vi "Teleop.vi"(0 "Call Context":T2, 1 "Match Info":T1={"Autonomous Elapsed Seconds"=0.0, "TeleOp Elapsed Seconds"=0.0, "Disabled Elapsed Seconds"=0.0, "Visited Autonomous"=FALSE, "Visited TeleOp"=FALSE, "Visited Disabled"=FALSE, "Autonomous Settings"={"Autonomous Style"=enum."Independent", "VI Refnum"=refnum}}) -> ()   [LabVIEW 2017]
doc: "This VI is called for each TeleOp packet received from the DS where the robot is not disabled. It is often used to read from the joysticks and update I/O or to update setpoints for timed control loops. It should complete and return within 20 milliseconds or it may miss DS packets."
uses:
  <vilib>/Rock Robotics/Network Tables/NT Write Numeric Array.vi
  <vilib>/Rock Robotics/Network Tables/NT Write Boolean Array.vi
  <vilib>/Rock Robotics/Network Tables/NT Read Boolean.vi
  <vilib>/Rock Robotics/Network Tables/NT Read Number.vi
  <vilib>/Rock Robotics/WPI/DriverStation/WPI_DriverStationMatch Info.ctl
  <vilib>/Rock Robotics/WPI/DriverStation/WPI_DriverStationDerivedRobotMode.ctl
panel:
  out "Compressor Running":bool
  out "Enabled":bool
  out "Sample Slider 0":dbl(slide) scale=0.0..5.0
  out "Sample Boolean 1":bool
  out "Sample Boolean 0":bool
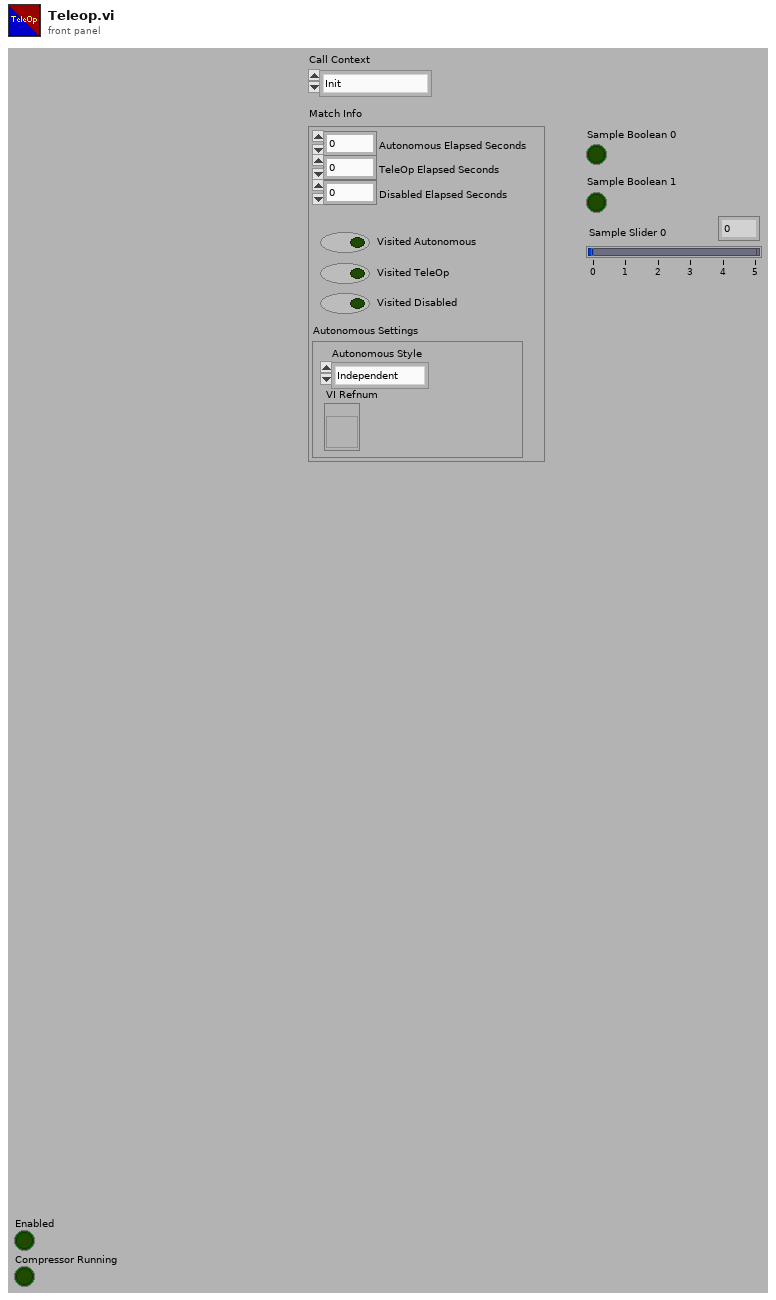
[diagram p1: front panel]
types:
  T1 = typedef "WPI_DriverStationMatch Info.ctl" = cluster{"Autonomous Elapsed Seconds":dbl, "TeleOp Elapsed Seconds":dbl, "Disabled Elapsed Seconds":dbl, "Visited Autonomous":bool, "Visited TeleOp":bool, "Visited Disabled":bool, "Autonomous Settings":cluster{"Autonomous Style":enum16{"Iterative", "Independent"}, "VI Refnum":refnum<vi>}}
  T2 = typedef "WPI_DriverStationDerivedRobotMode.ctl" = enum16{"Init", "Execute", "Stop"}
  T3 = typedef "WPI_CompressorDevRef.ctl" = cluster{"DevStatus":errorcluster, "Pneumatics Control Module":u8}
  T4 = typedef "WPI_JoystickDevRef.ctl" = cluster{"Device":T5}
  T5 = typedef "WPI_JoystickDeviceEnum.ctl" = enum16{"USB 0", "USB 1", "USB 2", "USB 3", "USB 4", "USB 5"}
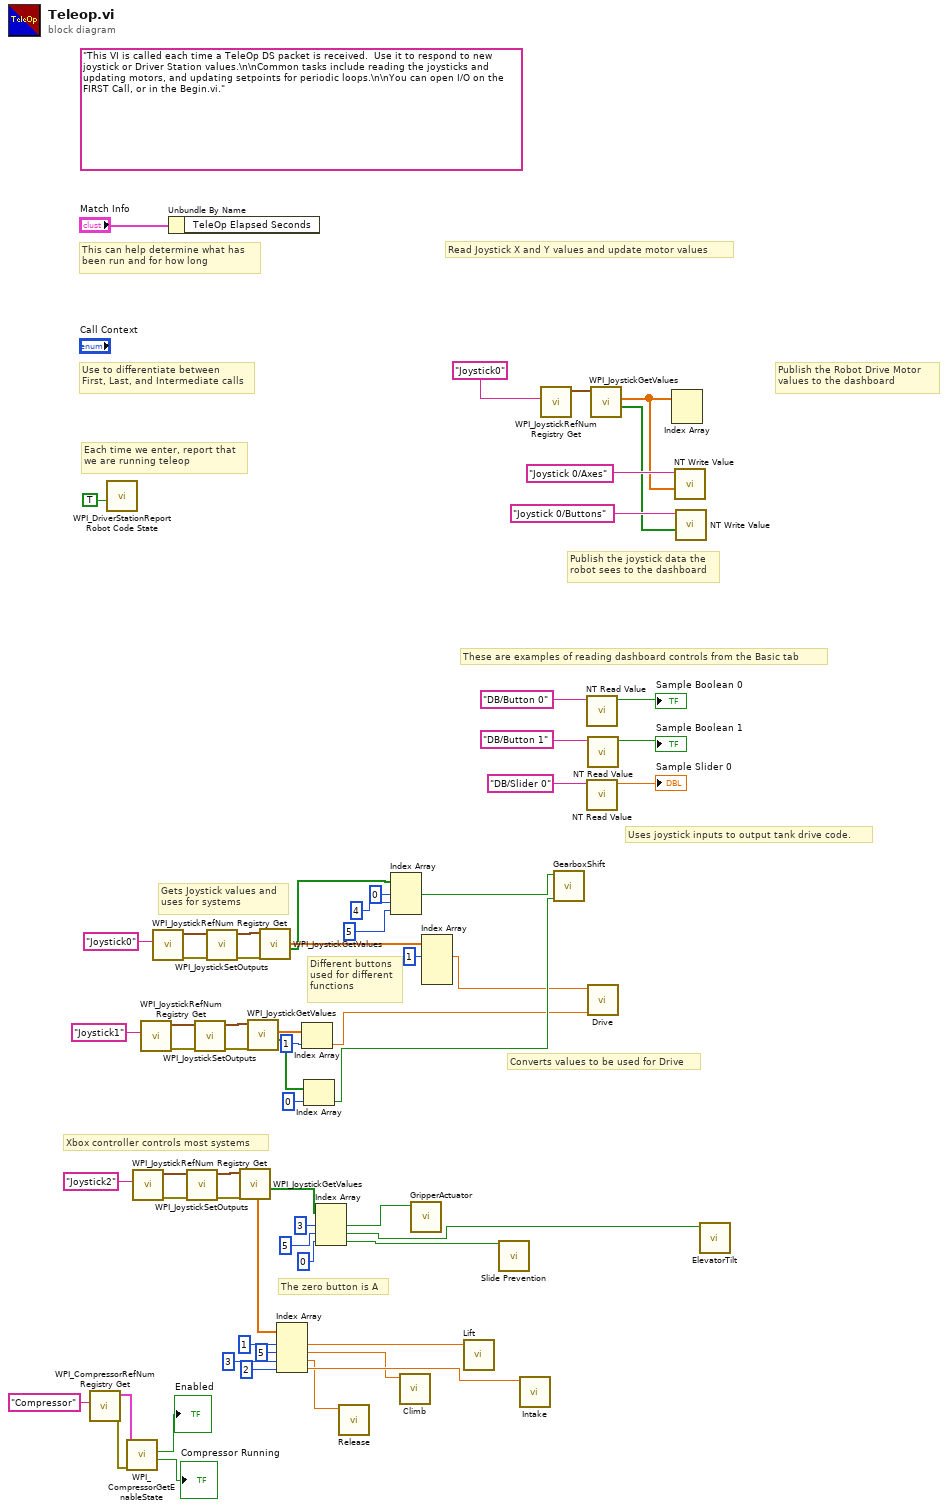
[diagram p0: block diagram]
diagram:
  (unwired) "This VI is called each time a TeleOp DS packet is received.  Use it to respond to new joystick or Driver Station values.\n\nCommon tasks include reading the joysticks and updating motors, and updating setpoints for periodic loops.\n\nYou can open I/O on the FIRST Call, or in the Begin.vi."
  # "The zero button is A"
  # "Xbox controller controls most systems"
  # "Converts values to be used for Drive"
  # "Different buttons\nused for different\nfunctions"
  # "Gets Joystick values and\nuses for systems"
  # "Uses joystick inputs to output tank drive code."
  # "These are examples of reading dashboard controls from the Basic tab"
  # "Publish the Robot Drive Motor\nvalues to the dashboard"
  # "Publish the joystick data the\nrobot sees to the dashboard"
  # "Each time we enter, report that\nwe are running teleop"
  # "Use to differentiate between\nFirst, Last, and Intermediate calls"
  # "This can help determine what has\nbeen run and for how long"
  # "Read Joystick X and Y values and update motor values"
  n1 = call <vilib>:"WPI_CompressorRefNum Registry Get.vi"("refnum name"="Compressor") -> ("error out"=w25:errorcluster, "CompressorDevRef"=w24:T3)  [unwired: 9 in]
  n2 = call <vilib>:"WPI_DriverStationReport Robot Code State.vi"("TeleOp"=TRUE ("Autonomous")) -> ()  [unwired: 10 in, 1 out]
  n3 = call <vilib>:"WPI_CompressorGetEnableState.vi"("error in (no error)"=w25, "CompressorDevRef"=w24) -> ("Compressor Running"=→"Compressor Running":bool, "Enabled"=→"Enabled":bool)  [unwired: 6 in, 2 out]
  n4 = call <vilib>:"WPI_JoystickRefNum Registry Get.vi"("refnum name"="Joystick2") -> ("error out"=w31:errorcluster, "JoystickDevRef"=w33:T4)  [unwired: 1 in, 8 out]
  n5 = call <vilib>:"WPI_JoystickRefNum Registry Get.vi"("refnum name"="Joystick1") -> ("error out"=w42:errorcluster, "JoystickDevRef"=w40:T4)  [unwired: 1 in, 8 out]
  n6 = call <vilib>:"WPI_JoystickRefNum Registry Get.vi"("refnum name"="Joystick0") -> ("error out"=w45:errorcluster, "JoystickDevRef"=w47:T4)  [unwired: 1 in, 8 out]
  n7 = Unbundle By Name("Match Info") -> ()  [unwired: 1 out]
  n8 = call <vilib>:"WPI_JoystickSetOutputs.vi"("error in (no error)"=w31, "JoystickDevRef"=w33) -> ("error out"=w30:errorcluster, "JoystickDevRef"=w32:T4)  [unwired: 8 in]
  n9 = call <vilib>:"WPI_JoystickSetOutputs.vi"("error in (no error)"=w42, "JoystickDevRef"=w40) -> ("error out"=w43:errorcluster, "JoystickDevRef"=w41:T4)  [unwired: 8 in]
  n10 = call <vilib>:"WPI_JoystickSetOutputs.vi"("error in (no error)"=w45, "JoystickDevRef"=w47) -> ("error out"=w44:errorcluster, "JoystickDevRef"=w46:T4)  [unwired: 8 in]
  n11 = call <vilib>:"WPI_JoystickGetValues.vi"("error in (no error)"=w30, "JoystickDevRef"=w32) -> ("Buttons"=w29:bool[], "Axes"=w26:dbl[])  [unwired: 5 in, 3 out]
  n12 = call <vilib>:"WPI_JoystickGetValues.vi"("error in (no error)"=w43, "JoystickDevRef"=w41) -> ("Buttons"=w19:bool[], "Axes"=w38:dbl[])  [unwired: 5 in, 3 out]
  n13 = call <vilib>:"WPI_JoystickGetValues.vi"("error in (no error)"=w44, "JoystickDevRef"=w46) -> ("Buttons"=w35:bool[], "Axes"=w50:dbl[])  [unwired: 5 in, 3 out]
  n14 = Index Array(array=w26, index #1=1 ("index"), index #2=5 ("index"), index #3=3 ("index"), index #4=2 ("index")) -> (element #1=w7:dbl, element #2=w5:dbl, element #3=w6:dbl, element #4=w8:dbl)
  n15 = Index Array(array=w38, index=1) -> (element=w15:dbl)
  n16 = Index Array(array=w19, index=0) -> (element=w17:bool)
  n17 = Index Array(array=w29, index #1=3 ("index"), index #2=5 ("index"), index #3=0 ("index")) -> (element #1=w10:bool, element #2=w4:bool, element #3=w1:bool)
  n18 = call "Release.vi"("Release"=w6) -> ()  [unwired: 11 in]
  n19 = Index Array(array=w35, index #1=0 ("index"), index #2=4 ("index"), index #3=5 ("index")) -> (element #1=w20:bool)  [unwired: 2 out]
  n20 = call "Climb.vi"("EFfort"=w5) -> ()  [unwired: 11 in]
  n21 = call "GripperActuator.vi"("Up"=w10) -> ()  [unwired: 11 in]
  n22 = Index Array(array=w50, index #1=1 ("index")) -> (element #1=w16:dbl)  [unwired: 3 in, 3 out]
  n23 = call "Lift.vi"("Effort"=w7) -> ()  [unwired: 11 in]
  n24 = call "Slide Prevention.vi"("Slide?"=w1) -> ()  [unwired: 11 in]
  n25 = call "Intake.vi"("Intake"=w8) -> ()  [unwired: 11 in]
  n26 = call <vilib>:"WPI_JoystickRefNum Registry Get.vi"("refnum name"="Joystick0") -> ("JoystickDevRef"=w62:T4)  [unwired: 1 in, 9 out]
  n27 = call "GearboxShift.vi"("Gear2"=w17, "Gear1"=w20) -> ()  [unwired: 10 in]
  n28 = call-poly <vilib>:"NT Read Value.vi"("Name"="DB/Button 0" ("refnum name")) -> ("Boolean"=→"Sample Boolean 0":bool)  [unwired: 9 in, 1 out]
  n29 = call-poly <vilib>:"NT Read Value.vi"("Name"="DB/Slider 0" ("refnum name")) -> ("Numeric"=→"Sample Slider 0":dbl)  [unwired: 9 in, 1 out]
  n30 = call-poly <vilib>:"NT Read Value.vi"("Name"="DB/Button 1" ("refnum name")) -> ("Boolean"=→"Sample Boolean 1":bool)  [unwired: 9 in, 1 out]
  n31 = call "Drive.vi"("Drive R"=w15, "Drive L"=w16) -> ()  [unwired: 10 in]
  n32 = call <vilib>:"WPI_JoystickGetValues.vi"("JoystickDevRef"=w62) -> ("Buttons"=w57:bool[], "Axes"=w58:dbl[])  [unwired: 6 in, 3 out]
  n33 = Index Array(array=w58) -> ()  [unwired: 2 in, 2 out]
  n34 = call-poly <vilib>:"NT Write Value.vi"("Numeric Array"=w58, "Name"="Joystick 0/Axes") -> ()  [unwired: 9 in, 1 out]
  n35 = call-poly <vilib>:"NT Write Value.vi"("Boolean Array"=w57, "Name"="Joystick 0/Buttons") -> ()  [unwired: 9 in, 1 out]
  n36 = call "ElevatorTilt.vi"("Up"=w4) -> ()  [unwired: 11 in]
